vi "Select Object for Registration.vi"() -> (0 "Side":T1=enum."right", 1 "Object":string, 3 "File":path)   [LabVIEW 2013]
uses:
  ROS/Code/SubVIs/BaxterSide.ctl
panel:
  in  "Done":bool
  in  "Listbox":i32(listbox)
  # "Select Object"
  # "Then Press DONE"
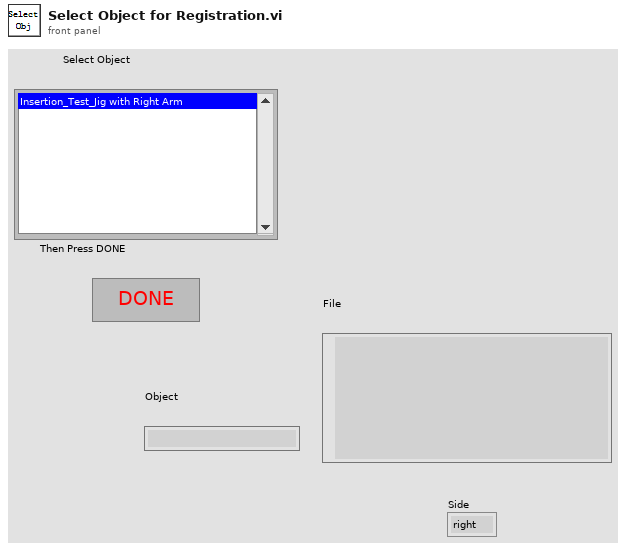
[diagram p1: front panel]
types:
  T1 = typedef "BaxterSide.ctl" = enum16{"left", "right"}
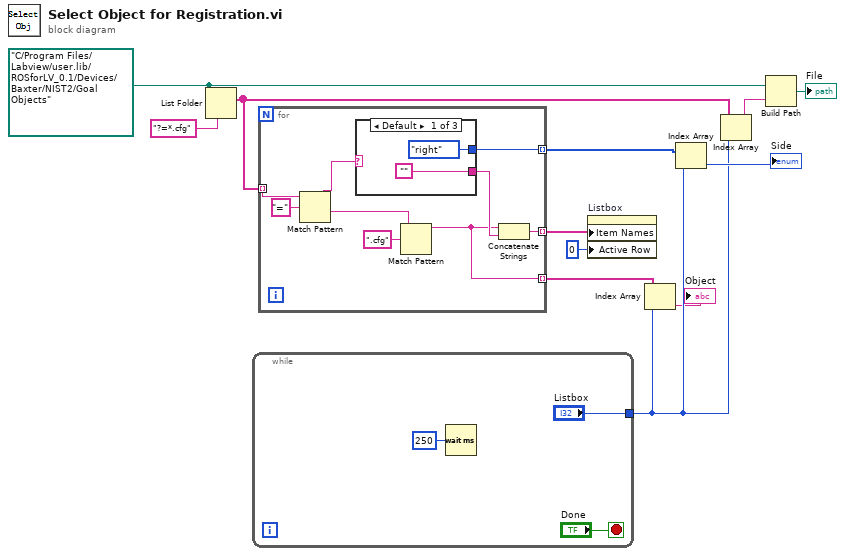
[diagram p0: block diagram]
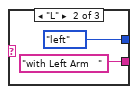
[diagram p2: hidden frame]
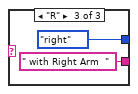
[diagram p3: hidden frame]
diagram:
  w8 = path "C:/Program Files/Labview/user.lib/ROSforLV_0.1/Devices/Baxter/NIST2/Goal Objects" ("base path")
  n1 = List Folder(path=w8, pattern="?=*.cfg") -> (filenames=w9:string[])  [unwired: 2 in, 3 out]
  n2 = while {
    tunnel: ["Listbox"] -> w2
    stop <- "Done" stop-if-true
    n3 = Wait (ms)(milliseconds to wait=u32 250) -> ()  [unwired: 1 out]
  }
  n4 = for {
    tunnel: w9 -> [w24] mode=indexing
    tunnel: [w19] -> w11 mode=indexing
    tunnel: [w17] -> w5 mode=indexing
    tunnel: [w16] -> w3 mode=indexing
    n5 = Match Pattern(string=w24, regular expression="=") -> (before substring=w22:string, after substring=w21:string)  [unwired: 1 in, 2 out]
    n6 = case shown="Default" w22 {
      tunnel: ["" "with Left Arm   " " with Right Arm  "] -> w18
      tunnel: [BaxterSide."right" ("Side") BaxterSide."left" ("Side") BaxterSide."right" ("Side")] -> w17
      frame Default {
      }
      frame "L" {
      }
      frame "R" {
      }
    }
    n7 = Match Pattern(string=w21, regular expression=".cfg") -> (before substring=w16:string)  [unwired: 1 in, 3 out]
    n8 = Concatenate Strings(w16, w18) -> (w19:string)
  }
  n9 = property on="Listbox" class="LstBox (strict)"("Item Names"=w11, "Active Row"=0 ("Active Row:Active Row Number")) -> ()  [unwired: 2 in, 2 out]
  n10 = Index Array(array=w3, index=w2) -> (element=→"Object":string)
  n11 = Index Array(array=w5, index=w2) -> (element=→"Side":T1)
  n12 = Index Array(array=w9, index=w2) -> (element=w7:string)
  n13 = Build Path(base path=w8, name or relative path=w7) -> (appended path=→"File":path)
